vi "DMARS_Frame_v2_write.vi"(11 "DMARS":dbl[](array[numeric])) -> (0 "No DMARS string":bool, 3 "string_Out":string)   [LabVIEW 2011]
panel:
  out "unsigned 32bit integer":u32
  out "SubFrame":u8
  out "sec":dbl
  out "size(s)":i32
  out "output array":u8[](array[numeric]) format="%x"
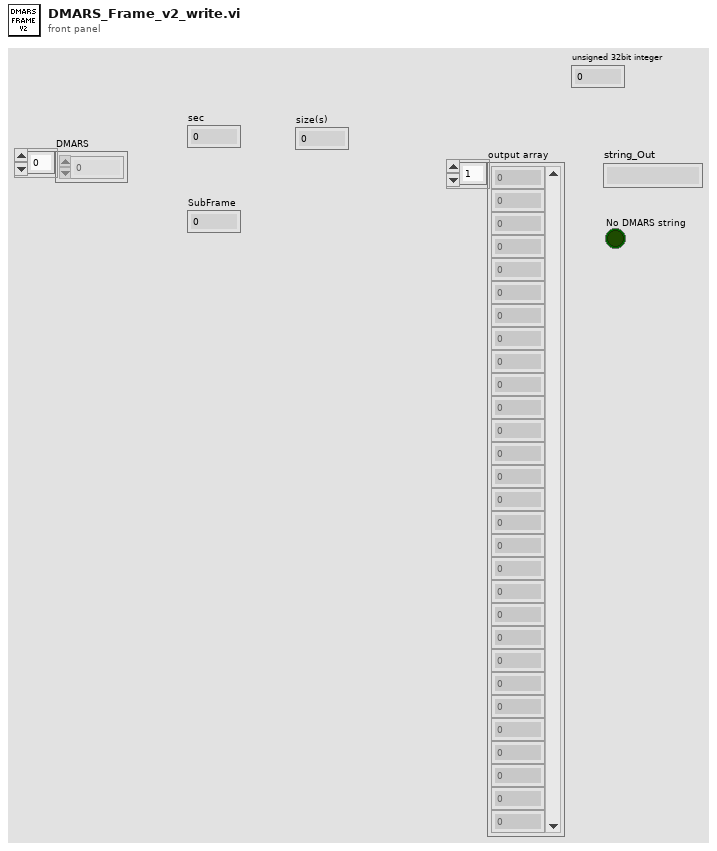
[diagram p1: front panel]
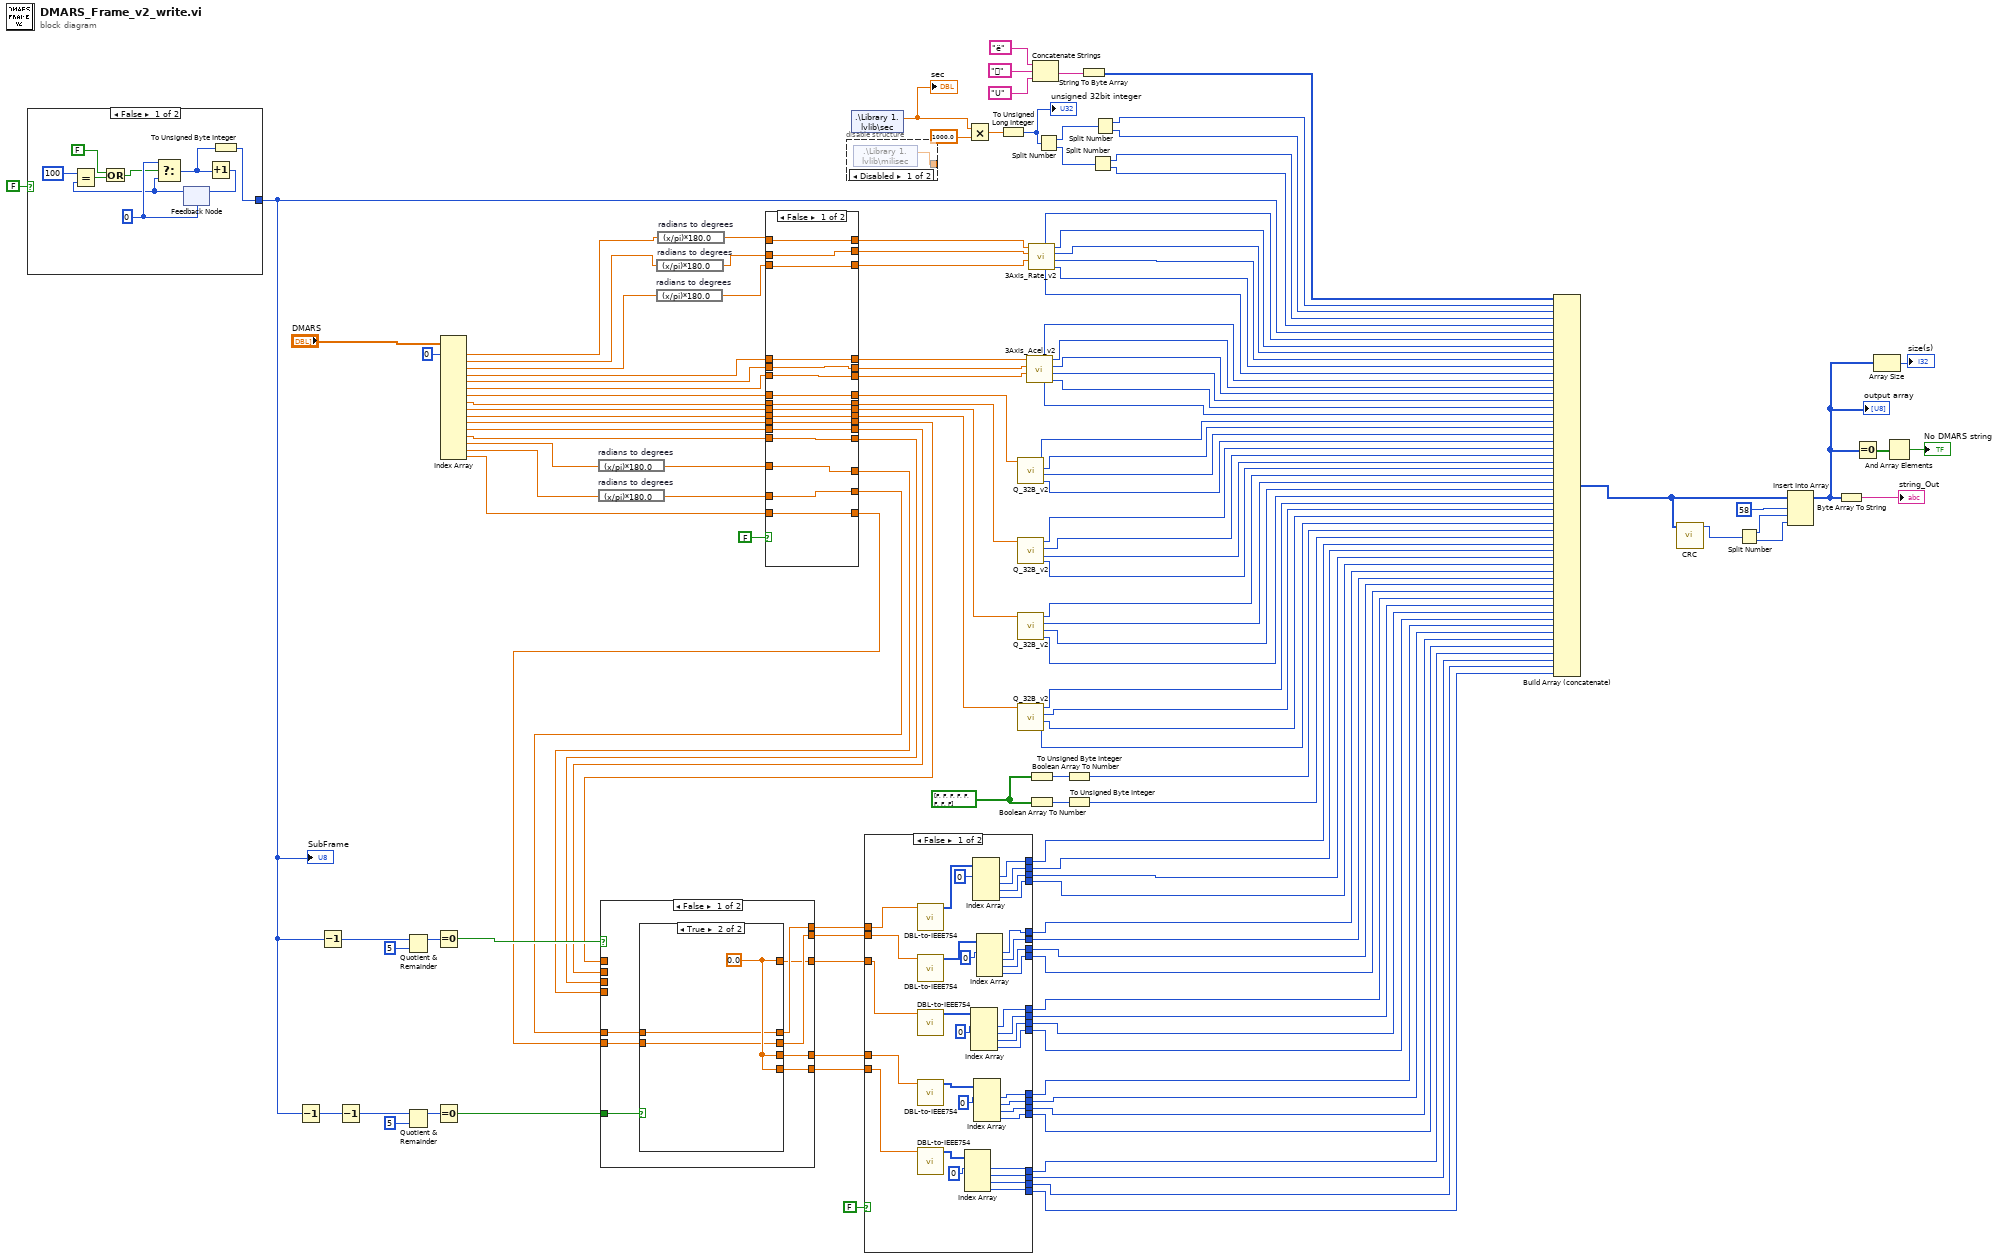
[diagram p0: block diagram]
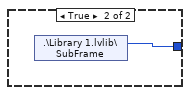
[diagram p2: hidden frame]
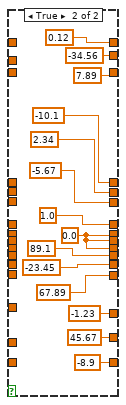
[diagram p4: hidden frame]
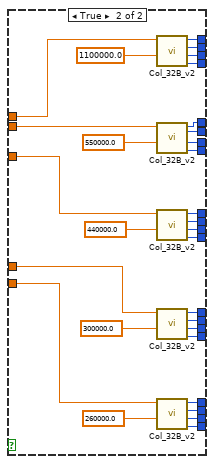
[diagram p5: hidden frame]
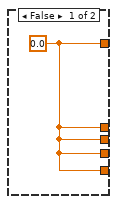
[diagram p6: hidden frame]
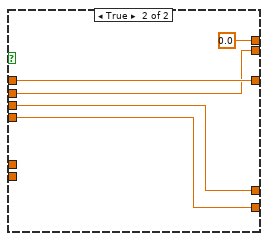
[diagram p7: hidden frame]
diagram:
  w69 = bool[] [FALSE, FALSE, FALSE, FALSE, FALSE, FALSE, FALSE, FALSE] ("Byte 36")
  n1 = case shown="False" FALSE {
    tunnel: [w137 w145] -> w59
    frame False {
      w144 = 0 ("x")
      n2 = feedback #1(w144) -> (w139:i32)
      n3 = Equal?(x=100, y=w139) -> (x = y?=w140:bool)
      n4 = Or(x=FALSE, y=w140) -> (x .or. y?=w141:bool)
      n5 = Select(t=w144, s=w141, f=w139) -> (s? t:f=w142:i32)
      n6 = Increment(x=w142) -> (x+1=w143:i32)
      n7 = feedback-in #1(w143) -> ()
      n8 = To Unsigned Byte Integer(number=w142) -> (unsigned 8bit integer=w137:u8)
    }
    frame True {
      n9 = shared-variable ".\\Library 1.lvlib\\SubFrame"() -> (w145:u8)  [unwired: 1 in, 1 out]
    }
  }
  "SubFrame" <- w59
  n10 = Decrement(x=w59) -> (x-1=w60:u8)
  n11 = Decrement(x=w59) -> (x-1=w64:u8)
  n12 = Decrement(x=w60) -> (x-1=w63:u8)
  n13 = Quotient & Remainder(x=w64, y=u8 5) -> (x-y*floor(x/y)=w66:u8)  [unwired: 1 out]
  n14 = Quotient & Remainder(x=w63, y=u8 5) -> (x-y*floor(x/y)=w62:u8)  [unwired: 1 out]
  n15 = Equal To 0?(x=w66) -> (x = 0?=w65:bool)
  n16 = Equal To 0?(x=w62) -> (x = 0?=w53:bool)
  n17 = Index Array(array="DMARS", index #1=0 ("index")) -> (element #1=w18:dbl, element #2=w16:dbl, element #3=w15:dbl, element #4=w44:dbl, element #5=w42:dbl, element #6=w40:dbl, element #7=w38:dbl, element #8=w36:dbl, element #9=w35:dbl, element #10=w32:dbl, element #11=w30:dbl, element #12=w28:dbl, element #13=w26:dbl, element #14=w52:dbl, element #15=w51:dbl, element #16=w20:dbl)  [unwired: 15 in]
  n18 = expression code="(x/pi)*180.0" "radians to degrees"(w52) -> (w24:dbl)
  n19 = expression code="(x/pi)*180.0" "radians to degrees"(w51) -> (w22:dbl)
  n20 = expression code="(x/pi)*180.0" "radians to degrees"(w15) -> (w13:dbl)
  n21 = expression code="(x/pi)*180.0" "radians to degrees"(w16) -> (w14:dbl)
  n22 = expression code="(x/pi)*180.0" "radians to degrees"(w18) -> (w17:dbl)
  n23 = case shown="False" FALSE {
    tunnel: [w161 0.12 ("Numeric")] -> w48
    tunnel: w17 -> [w161 _]
    tunnel: [w160 -34.56 ("Numeric")] -> w47
    tunnel: w14 -> [w160 _]
    tunnel: [w146 7.89 ("Numeric")] -> w46
    tunnel: w13 -> [w146 _]
    tunnel: [w159 -10.1 ("Numeric")] -> w45
    tunnel: w44 -> [w159 _]
    tunnel: [w158 2.34 ("Numeric")] -> w43
    tunnel: w42 -> [w158 _]
    tunnel: [w157 -5.67 ("Numeric")] -> w41
    tunnel: w40 -> [w157 _]
    tunnel: [w156 1.0 ("Numeric")] -> w39
    tunnel: w38 -> [w156 _]
    tunnel: [w155 w168] -> w37
    tunnel: w36 -> [w155 _]
    tunnel: w35 -> [w154 _]
    tunnel: [w154 w168] -> w34
    tunnel: [w153 w168] -> w33
    tunnel: w32 -> [w153 _]
    tunnel: [w152 89.1 ("Numeric")] -> w31
    tunnel: w30 -> [w152 _]
    tunnel: [w151 -23.45 ("Numeric")] -> w29
    tunnel: w28 -> [w151 _]
    tunnel: [w150 67.89 ("Numeric")] -> w27
    tunnel: w26 -> [w150 _]
    tunnel: [w149 -1.23 ("Numeric")] -> w25
    tunnel: w24 -> [w149 _]
    tunnel: [w148 45.67 ("Numeric")] -> w23
    tunnel: w22 -> [w148 _]
    tunnel: [w147 -8.9 ("Numeric")] -> w21
    tunnel: w20 -> [w147 _]
    frame False {
    }
    frame True {
      w168 = 0.0 ("Numeric")
    }
  }
  n24 = case shown="False" w65 {
    tunnel: w31 -> [_ w191]
    tunnel: w29 -> [_ w190]
    tunnel: w27 -> [_ w189]
    tunnel: w25 -> [_ w188]
    tunnel: [w180 0.0] -> w58
    tunnel: [w178 w191] -> w57
    tunnel: [w179 w190] -> w56
    tunnel: [w177 w189] -> w55
    tunnel: [w176 w188] -> w54
    tunnel: w53 -> [w183 _]
    tunnel: w23 -> [w182 _]
    tunnel: w21 -> [w181 _]
    frame False {
      n25 = case shown="True" w183 {
        tunnel: w182 -> [_ w186]
        tunnel: w181 -> [_ w185]
        tunnel: [w184 w186] -> w180
        tunnel: [w184 w185] -> w179
        tunnel: [w184 w187] -> w178
        tunnel: [w184 w187] -> w177
        tunnel: [w184 w187] -> w176
        frame False {
          w184 = 0.0
        }
        frame True {
          w187 = 0.0
        }
      }
    }
    frame True {
    }
  }
  n26 = disable-structure shown="Disabled" {
    disable-tunnel: [w193 _] -> _
    frame Disabled {
      n27 = shared-variable ".\\Library 1.lvlib\\milisec"() -> (w193:dbl)  [unwired: 1 in, 1 out]
    }
    frame Enabled {
    }
  }
  n28 = shared-variable ".\\Library 1.lvlib\\sec"() -> (w2:dbl)  [unwired: 1 in, 1 out]
  "sec" <- w2
  n29 = case shown="False" FALSE {
    tunnel: [w197 w258] -> w130
    tunnel: [w194 w257] -> w129
    tunnel: [w195 w256] -> w128
    tunnel: [w196 w255] -> w127
    tunnel: [w198 w254] -> w126
    tunnel: [w199 w253] -> w125
    tunnel: [w200 w252] -> w124
    tunnel: [w201 w251] -> w123
    tunnel: [w206 w250] -> w122
    tunnel: [w207 w249] -> w121
    tunnel: [w208 w248] -> w120
    tunnel: [w209 w247] -> w119
    tunnel: [w212 w246] -> w118
    tunnel: [w213 w245] -> w117
    tunnel: [w214 w244] -> w116
    tunnel: [w215 w243] -> w115
    tunnel: [w219 w242] -> w114
    tunnel: [w220 w241] -> w113
    tunnel: [w221 w240] -> w112
    tunnel: [w222 w239] -> w111
    tunnel: w58 -> [w228 w238]
    tunnel: w57 -> [w226 w237]
    tunnel: w56 -> [w227 w236]
    tunnel: w55 -> [w225 w235]
    tunnel: w54 -> [w224 w234]
    frame False {
      n30 = call "DBL-to-IEEE754.vi"("Input_DBL"=w228) -> ("Output_U8"=w223:u8[])  [unwired: 10 in]
      n31 = call "DBL-to-IEEE754.vi"("Input_DBL"=w227) -> ("Output_U8"=w217:u8[])  [unwired: 10 in]
      n32 = call "DBL-to-IEEE754.vi"("Input_DBL"=w226) -> ("Output_U8"=w210:u8[])  [unwired: 10 in]
      n33 = call "DBL-to-IEEE754.vi"("Input_DBL"=w225) -> ("Output_U8"=w202:u8[])  [unwired: 10 in]
      n34 = call "DBL-to-IEEE754.vi"("Input_DBL"=w224) -> ("Output_U8"=w203:u8[])  [unwired: 10 in]
      n35 = Index Array(array=w203, index #1=0 ("index")) -> (element #1=w197:u8, element #2=w196:u8, element #3=w195:u8, element #4=w194:u8)  [unwired: 3 in]
      n36 = Index Array(array=w210, index #1=0 ("index")) -> (element #1=w209:u8, element #2=w208:u8, element #3=w207:u8, element #4=w206:u8)  [unwired: 3 in]
      n37 = Index Array(array=w223, index #1=0 ("index")) -> (element #1=w222:u8, element #2=w221:u8, element #3=w220:u8, element #4=w219:u8)  [unwired: 3 in]
      n38 = Index Array(array=w202, index #1=0 ("index")) -> (element #1=w201:u8, element #2=w200:u8, element #3=w199:u8, element #4=w198:u8)  [unwired: 3 in]
      n39 = Index Array(array=w217, index #1=0 ("index")) -> (element #1=w215:u8, element #2=w214:u8, element #3=w213:u8, element #4=w212:u8)  [unwired: 3 in]
    }
    frame True {
      n40 = call "Col_32B_v2.vi"("Ref"=1100000.0, "Col"=w238) -> ("LL"=w242:u8, "LH"=w241:u8, "HL"=w240:u8, "HH"=w239:u8)  [unwired: 6 in]
      n41 = call "Col_32B_v2.vi"("Ref"=550000.0, "Col"=w236) -> ("LL"=w246:u8, "LH"=w245:u8, "HL"=w244:u8, "HH"=w243:u8)  [unwired: 6 in]
      n42 = call "Col_32B_v2.vi"("Ref"=440000.0, "Col"=w237) -> ("LL"=w250:u8, "LH"=w249:u8, "HL"=w248:u8, "HH"=w247:u8)  [unwired: 6 in]
      n43 = call "Col_32B_v2.vi"("Ref"=300000.0, "Col"=w235) -> ("LL"=w254:u8, "LH"=w253:u8, "HL"=w252:u8, "HH"=w251:u8)  [unwired: 6 in]
      n44 = call "Col_32B_v2.vi"("Ref"=260000.0, "Col"=w234) -> ("LL"=w257:u8, "LH"=w256:u8, "HL"=w255:u8, "HH"=w258:u8)  [unwired: 6 in]
    }
  }
  n45 = Multiply(x=w2, y=1000.0) -> (x*y=w3:dbl)
  n46 = To Unsigned Long Integer(number=w3) -> (unsigned 32bit integer=w7:u32)
  "unsigned 32bit integer" <- w7
  n47 = call "Q_32B_v2.vi"("Q_32B"=w39) -> ("LL"=w96:u8, "HL"=w95:u8, "LH"=w94:u8, "HH"=w93:u8)  [unwired: 7 in]
  n48 = call "Q_32B_v2.vi"("Q_32B"=w37) -> ("LL"=w100:u8, "HL"=w99:u8, "LH"=w98:u8, "HH"=w97:u8)  [unwired: 7 in]
  n49 = call "Q_32B_v2.vi"("Q_32B"=w34) -> ("LL"=w104:u8, "HL"=w103:u8, "LH"=w102:u8, "HH"=w101:u8)  [unwired: 7 in]
  n50 = call "Q_32B_v2.vi"("Q_32B"=w33) -> ("LL"=w108:u8, "HL"=w107:u8, "LH"=w106:u8, "HH"=w105:u8)  [unwired: 7 in]
  n51 = call "3Axis_Acel_v2.vi"("Roll_A"=w41, "Yaw_A"=w43, "Pitch_A"=w45) -> ("RAH"=w91:u8, "YAL"=w90:u8, "YAH"=w89:u8, "PAL"=w88:u8, "RAL"=w92:u8, "PAH"=w87:u8)  [unwired: 3 in]
  n52 = call "3Axis_Rate_v2.vi"("Roll_R"=w46, "Yaw_R"=w47, "Pitch_R"=w48) -> ("RRH"=w85:u8, "YRL"=w84:u8, "YRH"=w83:u8, "PRL"=w82:u8, "RRL"=w86:u8, "PRH"=w81:u8)  [unwired: 3 in]
  n53 = Boolean Array To Number(Boolean array=w69) -> (number=w79:u32)
  n54 = Boolean Array To Number(Boolean array=w69) -> (number=w78:u32)
  n55 = Concatenate Strings("ë", "", "U") -> (w74:string)
  n56 = Split Number(x=w7) -> (hi(x)=w6:u16, lo(x)=w5:u16)
  n57 = To Unsigned Byte Integer(number=w79) -> (unsigned 8bit integer=w109:u8)
  n58 = To Unsigned Byte Integer(number=w78) -> (unsigned 8bit integer=w110:u8)
  n59 = String To Byte Array(string=w74) -> (unsigned byte array=w80:u8[])
  n60 = Split Number(x=w5) -> (hi(x)=w132:u8, lo(x)=w133:u8)
  n61 = Split Number(x=w6) -> (hi(x)=w134:u8, lo(x)=w135:u8)
  n62 = Build Array (concatenate)(w80, w134, w135, w132, w133, w59, w81, w82, w83, w84, w85, w86, w87, w88, w89, w90, w91, w92, w93, w94, w95, w96, w97, w98, w99, w100, w101, w102, w103, w104, w105, w106, w107, w108, w109, w110, w111, w112, w113, w114, w115, w116, w117, w118, w119, w120, w121, w122, w123, w124, w125, w126, w130, w127, w128, w129) -> (w9:u8[])
  n63 = call "CRC.vi"("Array"=w9) -> ("CRC"=w8:u16)  [unwired: 10 in]
  n64 = Split Number(x=w8) -> (hi(x)=w72:u8, lo(x)=w71:u8)
  n65 = Insert Into Array(array=w9, index=58, new element #1=w72, new element #2=w71) -> (w12:u8[])
  "output array" <- w12
  n66 = Byte Array To String(unsigned byte array=w12) -> (string=→"string_Out":string)
  n67 = Equal To 0?(x=w12) -> (x = 0?=w11:bool[])
  n68 = Array Size(array=w12) -> (size(s)=→"size(s)":i32)
  n69 = And Array Elements(Boolean array=w11) -> (logical AND=→"No DMARS string":bool)
